vi "加载show.vi"(8 "error in (no error)":errorcluster caption="错误输入（无错误）") -> (0 "error out":errorcluster caption="错误输出")   [LabVIEW 2014]
doc: "该模板用于创建子VI。"
uses:
  <vilib>/Utility/config.llb/Read Key (String).vi
  glb/glb_data.vi
  <vilib>/Utility/config.llb/NI_LVConfig.lvlib
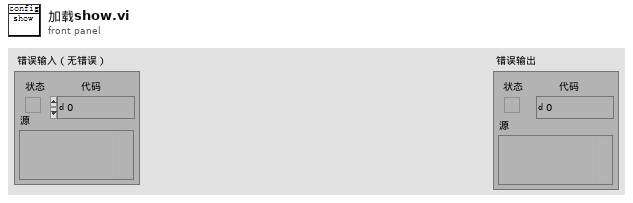
[diagram p1: front panel]
types:
  T1 = typedef "NI_LVConfig.lvlib/Config Data RefNum.ctl" = refnum<k1>
  T2 = cluster{"应用1":string[], "应用2":string[], "应用3":string[], "应用4":string[], "应用5":string[], "应用6":string[], "应用7":string[], "应用8":string[], "分母":cluster{"来源":string, "名称":string}, "加":cluster{"来源":string, "名称":string}[], "减":cluster{"来源":string, "名称":string}[]}
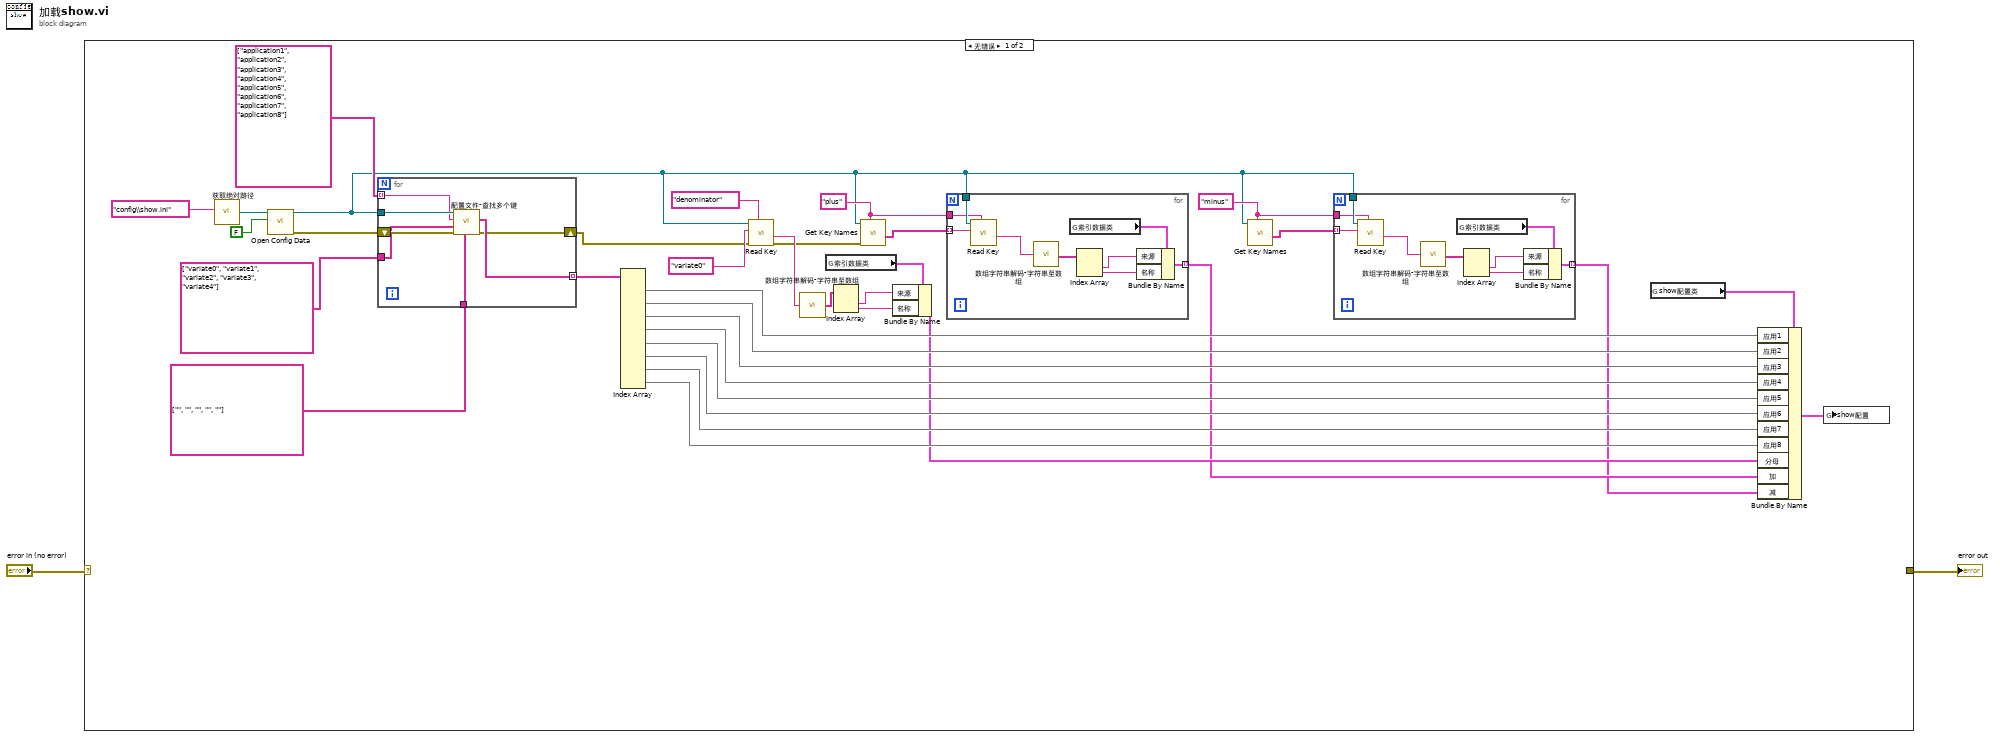
[diagram p0: block diagram]
diagram:
  n1 = case shown="无错误" "error in (no error)" {
    selector: "error in (no error)" -> [_ w63]
    tunnel: [_ w63] -> w1
    frame No Error {
      w22 = "minus" ("key")
      w23 = "plus" ("key")
      n2 = call "获取绝对路径.vi"("relativePath"="config\\show.ini" ("测试模块配置文件")) -> ("absolutePath"=w37:path)
      n3 = call <vilib>:"Open Config Data.vi"("create file if necessary (T)"=FALSE, "configuration file path"=w37) -> ("error out"=w34:errorcluster, "refnum"=w20:T1)  [unwired: 7 in, 1 out]
      n4 = for {
        tunnel: w20 -> [w62]
        tunnel: string[] ["application1", "application2", "application3", "application4", "application5", "application6", "application7", "application8"] -> [w60] mode=indexing
        tunnel: string[] ["variate0", "variate1", "variate2", "variate3", "variate4"] -> [w58]
        tunnel: string[] ["", "", "", "", ""] -> [w59]
        tunnel: [w57] -> w30 mode=indexing
        shift-right: [w56] -> w26
        shift-left: w34 -> [w61]
        n5 = call "配置文件-查找多个键.vi"("默认值"=w59, "错误输入（无错误）"=w61, "键名"=w58, "章名"=w60, "引用句柄输入"=w62) -> ("错误输出"=w56:errorcluster, "查询结果"=w57:string[])  [unwired: 4 in, 1 out]
      }
      n6 = Index Array(array=w30) -> (element #1=w18:string[], element #2=w17:string[], element #3=w16:string[], element #4=w15:string[], element #5=w14:string[], element #6=w13:string[], element #7=w12:string[], element #8=w11:string[])  [unwired: 16 in]
      n7 = call-poly <vilib>:"Read Key.vi"("section"="denominator" ("key"), "error in (no error)"=w26, "key"="variate0", "refnum"=w20) -> ("error out"=w25:errorcluster, "value"=w27:string)  [unwired: 4 in, 2 out]
      n8 = call "数组字符串解码-字符串至数组.vi"("字符串"=w27) -> ("数组"=w7:string[])  [unwired: 1 in]
      n9 = global read "类信息.vi" "索引数据类"() -> (w8:cluster{"来源":string, "名称":string})
      n10 = Index Array(array=w7) -> (element #1=w9:string, element #2=w10:string)  [unwired: 2 in]
      n11 = call <vilib>:"Get Key Names.vi"("section"=w23, "error in (no error)"=w25, "refnum"=w20) -> ("key names"=w24:string[])  [unwired: 5 in, 3 out]
      n12 = Bundle By Name(cluster=w8, "来源"=w9, "名称"=w10) -> (w6:cluster{"来源":string, "名称":string})
      n13 = for {
        tunnel: w20 -> [w55]
        tunnel: w24 -> [w54] mode=indexing
        tunnel: w23 -> [w53]
        tunnel: [w47] -> w5 mode=indexing
        n14 = call-poly <vilib>:"Read Key.vi"("section"=w53, "key"=w54, "refnum"=w55) -> ("value"=w52:string)  [unwired: 5 in, 3 out]
        n15 = call "数组字符串解码-字符串至数组.vi"("字符串"=w52) -> ("数组"=w51:string[])  [unwired: 1 in]
        n16 = global read "类信息.vi" "索引数据类"() -> (w50:cluster{"来源":string, "名称":string})
        n17 = Index Array(array=w51) -> (element #1=w49:string, element #2=w48:string)  [unwired: 2 in]
        n18 = Bundle By Name(cluster=w50, "来源"=w49, "名称"=w48) -> (w47:cluster{"来源":string, "名称":string})
      }
      n19 = call <vilib>:"Get Key Names.vi"("section"=w22, "refnum"=w20) -> ("key names"=w21:string[])  [unwired: 6 in, 3 out]
      n20 = for {
        tunnel: w20 -> [w46]
        tunnel: w21 -> [w45] mode=indexing
        tunnel: w22 -> [w44]
        tunnel: [w38] -> w4 mode=indexing
        n21 = call-poly <vilib>:"Read Key.vi"("section"=w44, "key"=w45, "refnum"=w46) -> ("value"=w43:string)  [unwired: 5 in, 3 out]
        n22 = call "数组字符串解码-字符串至数组.vi"("字符串"=w43) -> ("数组"=w42:string[])  [unwired: 1 in]
        n23 = global read "类信息.vi" "索引数据类"() -> (w41:cluster{"来源":string, "名称":string})
        n24 = Index Array(array=w42) -> (element #1=w40:string, element #2=w39:string)  [unwired: 2 in]
        n25 = Bundle By Name(cluster=w41, "来源"=w40, "名称"=w39) -> (w38:cluster{"来源":string, "名称":string})
      }
      n26 = global read "类信息.vi" "show配置类"() -> (w19:T2)
      n27 = Bundle By Name(cluster=w19, "应用1"=w18, "应用2"=w17, "应用3"=w16, "应用4"=w15, "应用5"=w14, "应用6"=w13, "应用7"=w12, "应用8"=w11, "分母"=w6, "加"=w5, "减"=w4) -> (w3:T2)
      n28 = global write "glb_data.vi" "show配置"(w3) -> ()
    }
    frame Error {
    }
  }
  "error out" <- w1
